vi "Rename Tag.vi"(7 "Prevent Overwrite? (F)":bool, 8 "error in (no error)":errorcluster, 9 "rename":string, 10 "tag":string, 11 "uData in":refnum<class "uData.lvclass">) -> (0 "error out":errorcluster, 1 "New Tag Replaced?":bool, 2 "Old Tag Found?":bool, 3 "uData out":refnum<class "uData.lvclass">)   [LabVIEW 2021, in "uData.lvlib" / "uData.lvclass"]
doc: "Rename an exiting tag. This will delete the old tag name and create a new tag name with the same payload data.\n\nThe 'new tag replaced' boolean returns a true if the new tag name already preexists."
uses:
  uData.lvclass
  uData.lvclass/uData.ctl
  Inline Replace Core.vi
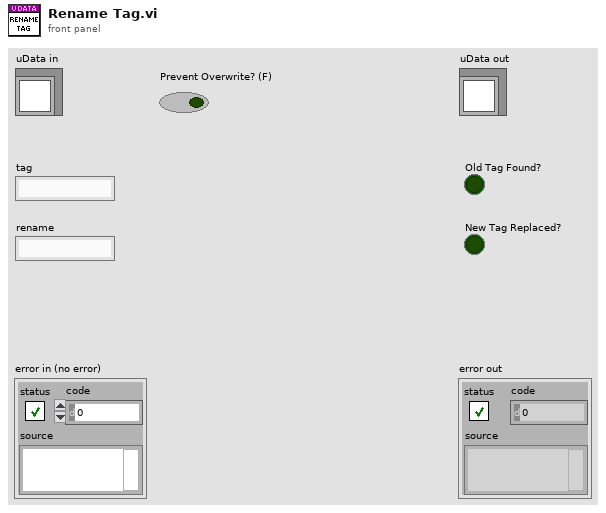
[diagram p1: front panel]
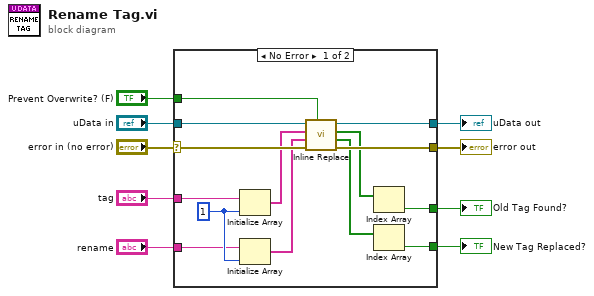
[diagram p0: block diagram]
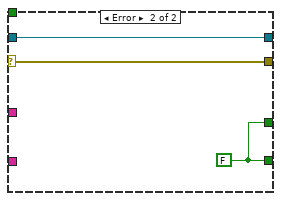
[diagram p2: hidden frame]
diagram:
  n1 = case shown="No Error" "error in (no error)" {
    selector: "error in (no error)" -> [w22 w26]
    tunnel: "uData in" -> [w21 w25]
    tunnel: [w20 w25] -> w9
    tunnel: [w23 w26] -> w8
    tunnel: "tag" -> [w17 _]
    tunnel: "rename" -> [w15 _]
    tunnel: [w14 w24] -> w4
    tunnel: [w12 w24] -> w3
    tunnel: "Prevent Overwrite? (F)" -> [w11 _]
    frame No Error {
      w18 = 1 ("dimension size")
      n2 = Initialize Array(w17, w18) -> (w16:string[])
      n3 = Initialize Array(w15, w18) -> (w10:string[])
      n4 = call "Inline Replace.vi"("Prevent Overwrite? (F)"=w11, "error in (no error)"=w22, "renamed keys"=w10, "keys"=w16, "uData in"=w21) -> ("error out"=w23:errorcluster, "replaced?"=w19:bool[], "Found?"=w13:bool[], "uData out"=w20:refnum<class "uData.lvclass">)  [unwired: 3 in]
      n5 = Index Array(array=w13) -> (element=w12:bool)  [unwired: 1 in]
      n6 = Index Array(array=w19) -> (element=w14:bool)  [unwired: 1 in]
    }
    frame Error {
      w24 = FALSE ("replaced")
    }
  }
  "error out" <- w8
  "uData out" <- w9
  "Old Tag Found?" <- w3
  "New Tag Replaced?" <- w4
